vi "CheckRunning.vi"(8 "error in (no error)":errorcluster, 11 "VISA resource name":refnum<visa-resource-name>) -> (0 "error out":errorcluster, 2 "IsRunning":bool, 3 "VISA resource name out":refnum<visa-resource-name>)   [LabVIEW 2009]
uses:
  Packet.ctl
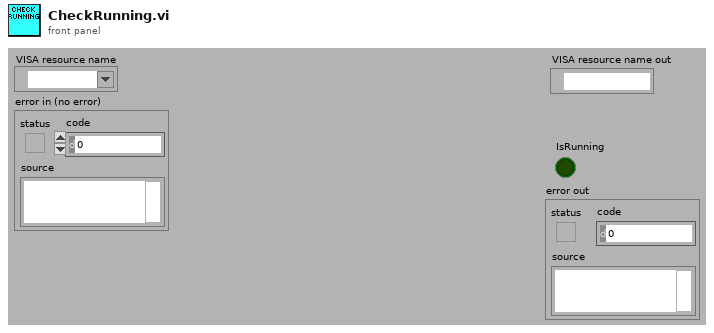
[diagram p1: front panel]
types:
  T1 = typedef "Packet.ctl" = cluster{"Length":u8, "Type":u8, "PID":u8, "Data":u8[], "CRC":u8}
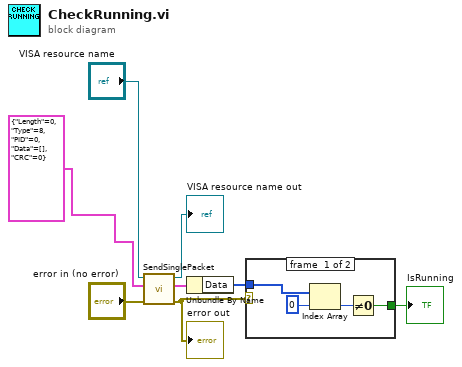
[diagram p0: block diagram]
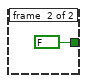
[diagram p2: hidden frame]
diagram:
  n1 = call "SendSinglePacket.vi"("error in (no error)"="error in (no error)", "Transmit"=T1 {"Length"=0, "Type"=8, "PID"=0, "Data"=[], "CRC"=0}, "VISA resource name"="VISA resource name") -> ("error out"=w2:errorcluster, "element"=w3:T1, "VISA resource name out"=→"VISA resource name out":refnum<visa-resource-name>)  [unwired: 6 in]
  "error out" <- w2
  n2 = Unbundle By Name(w3) -> ("Data"=w7:u8[])
  n3 = case shown="Error" w2 {
    tunnel: [w9 FALSE ("IsRunning")] -> w8
    tunnel: w7 -> [w12 _]
    frame #0 {
      n4 = Index Array(array=w12, index=0) -> (element=w10:u8)
      n5 = Not Equal To 0?(x=w10) -> (x != 0?=w9:bool)
    }
    frame #1 {
    }
  }
  "IsRunning" <- w8
